vi "Load Vendors.vi"(3 "errorIN":errorcluster, 5 "querySampleVendor":refnum<vi>) -> (0 "error OUT":errorcluster, 2 "Vendors":string[](array[string]))   [LabVIEW 2010]
uses:
  BIMS_Collector Globals.vi
panel:
  in  "lookup table name":string="SampleVendors"
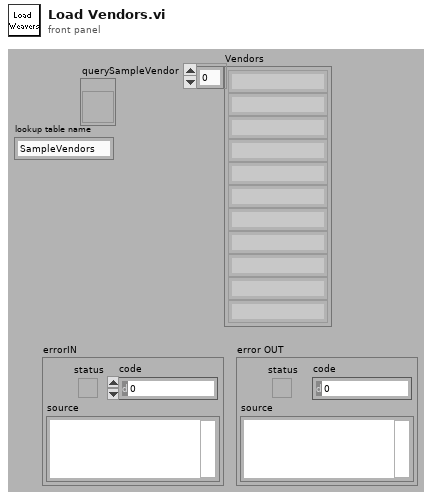
[diagram p1: front panel]
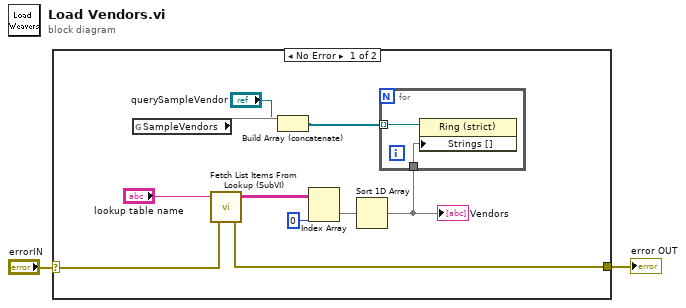
[diagram p0: block diagram]
diagram:
  n1 = case shown="No Error" "errorIN" {
    selector: "errorIN" -> [w8 w15]
    tunnel: [w7 w15] -> w2
    frame No Error {
      n2 = global read "BIMS_Collector Globals.vi" "SampleVendors"() -> (w5)
      n3 = call "Fetch List Items From Lookup (SubVI).vi"("error IN"=w8, "Query"="lookup table name") -> ("error OUT"=w7:errorcluster, "recordset data"=w12:string[][])  [unwired: 2 out]
      n4 = Build Array (concatenate)("querySampleVendor", w5) -> (w3:refnum<vi>[])
      n5 = Index Array(array=w12, index (col)=0 ("disabled index (col)")) -> (element=w10:string[])  [unwired: 1 in]
      n6 = Sort 1D Array(array=w10) -> (sorted array=w9:string[])
      "Vendors" <- w9
      n7 = for {
        tunnel: w3 -> [w14] mode=indexing
        tunnel: w9 -> [w13]
        n8 = property class="Ring (strict)"(reference=w14, "Strings []"=w13) -> ()  [unwired: 1 in, 2 out]
      }
    }
    frame Error {
    }
  }
  "error OUT" <- w2
